vi "Find project reference.vi"(3 "error in":errorcluster) -> (4 "ProjectName":T1=enum."SPIM", 5 "Sucess?":bool, 6 ".lvproj Filepath":path, 7 "Project Refnum":refnum<vi>, 8 "error out":errorcluster)   [LabVIEW 2013]
doc: "This .vi searches for the project in memory. This done by searching the projects in memory for one that matches this one. The appropriate ProjectName project conditional disable item must be present for the project, and a matching tag in the \"Check if current project\" subvi."
uses:
  File IO/Config/ProjectName enum.ctl
  Utility/Utility Lib.lvlib
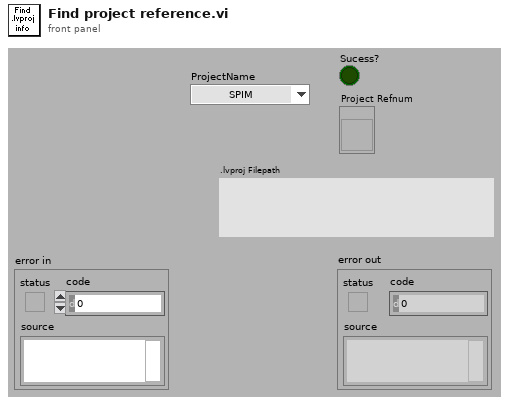
[diagram p1: front panel]
types:
  T1 = typedef "ProjectName enum.ctl" = enum16{"V-SIM", "SPIM", "TEMca2", "undefined", "HHMI Panels", "Wing Beat Analyzer"}
  T2 = enum32{"invalid app kind", "Development System", "Run Time System", "Student Edition", "Embedded LabVIEW", "Evaluation", "Custom"}
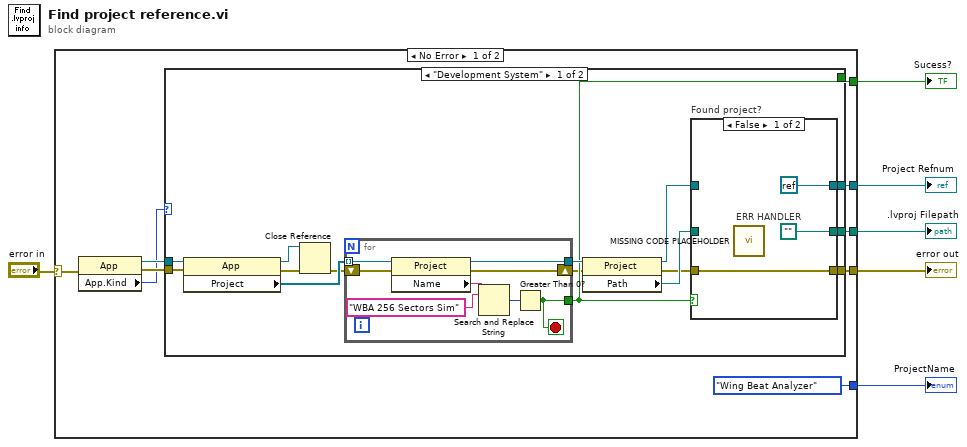
[diagram p0: block diagram]
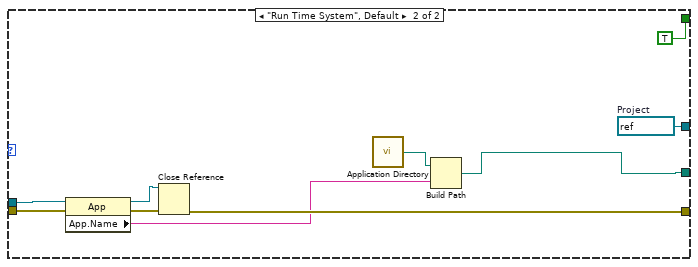
[diagram p3: hidden frame]
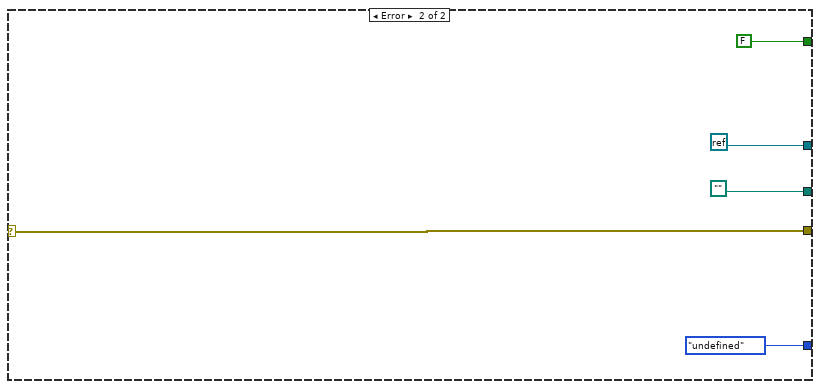
[diagram p4: hidden frame]
diagram:
  n1 = case shown="No Error" "error in" {
    selector: "error in" -> [w11 w59]
    tunnel: [w15 refnum<k0> refnum] -> w6
    tunnel: [w14 path ""] -> w5
    tunnel: [ProjectName_enum."Wing Beat Analyzer" ("ProjectName") ProjectName_enum."undefined" ("ProjectName")] -> w4
    tunnel: [w12 FALSE] -> w3
    tunnel: [w13 w59] -> w2
    frame No Error {
      n2 = property class="App"(error in=w11) -> (reference out=w9:refnum<vi>, error out=w10:errorcluster, "App.Kind"=w8:T2)  [unwired: 1 in]
      n3 = case shown="\"Development System\"" w8 {
        tunnel: [w30 w54] -> w15
        tunnel: [w29 w45] -> w14
        tunnel: [w24 w53] -> w13
        tunnel: [w19 TRUE] -> w12
        tunnel: w10 -> [w17 w50]
        tunnel: w9 -> [w16 w51]
        frame "Development System" {
          n4 = property class="App"(reference=w16, error in=w17) -> (reference out=w25:refnum<vi>, error out=w26:errorcluster, "Project"=w22:refnum<vi>[])
          n5 = Close Reference(reference=w25, error in (no error)=w26) -> (error out=w21:errorcluster)
          n6 = for {
            tunnel: w22 -> [w38] mode=indexing
            shift-right: [w34] -> w18
            shift-left: w21 -> [w37]
            tunnel: [w33] -> w20
            tunnel: [w31] -> w19
            stop <- w31 stop-if-true
            n7 = property class="Project"(reference=w38, error in=w37) -> (reference out=w33:refnum<vi>, error out=w34:errorcluster, "Name"=w36:string)
            n8 = Search and Replace String(input string=w36, search string="WBA 256 Sectors Sim") -> (number of replacements=w32:i32)  [unwired: 6 in, 3 out]
            n9 = Greater Than 0?(x=w32) -> (x > 0?=w31:bool)
          }
          n10 = property class="Project"(reference=w20, error in=w18) -> (reference out=w28:refnum<vi>, error out=w23:errorcluster, "Path"=w27:path)
          n11 = case "Found project?" shown="False" w19 {
            tunnel: w28 -> [_ w44]
            tunnel: [refnum<k0> refnum w44] -> w30
            tunnel: [path "" w43] -> w29
            tunnel: w27 -> [_ w43]
            tunnel: [w39 w42] -> w24
            tunnel: w23 -> [w39 w42]
            frame False {
              # "ERR HANDLER"
              n12 = call "MISSING CODE PLACEHOLDER.vi"() -> ()  [unwired: 1 in]
            }
            frame True {
            }
          }
        }
        frame "Run Time System", Default {
          w54 = refnum<vi> refnum  # Project
          n13 = property class="App"(reference=w51, error in=w50) -> (reference out=w47:refnum<vi>, error out=w48:errorcluster, "App.Name"=w49:string)
          n14 = Close Reference(reference=w47, error in (no error)=w48) -> (error out=w53:errorcluster)
          n15 = call <vilib>:"Application Directory.vi"() -> ("Application Directory"=w46:path)
          n16 = Build Path(base path=w46, name or relative path=w49) -> (appended path=w45:path)
        }
      }
    }
    frame Error {
    }
  }
  "error out" <- w2
  "Project Refnum" <- w6
  ".lvproj Filepath" <- w5
  "ProjectName" <- w4
  "Sucess?" <- w3
